vi "Drive Set Feet.vi"(1 "Feet":dbl=10.0 format="%#_13g", 2 "Direction":T1(ring)) -> (0 "Distance (ft)":dbl(knob) scale=0.0..10.0)   [LabVIEW 2014]
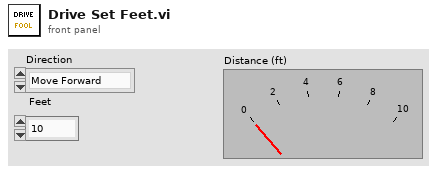
[diagram p1: front panel]
types:
  T1 = enum16{"Move Forward", "Move Backward", "Strafe Right", "Strafe Left"}
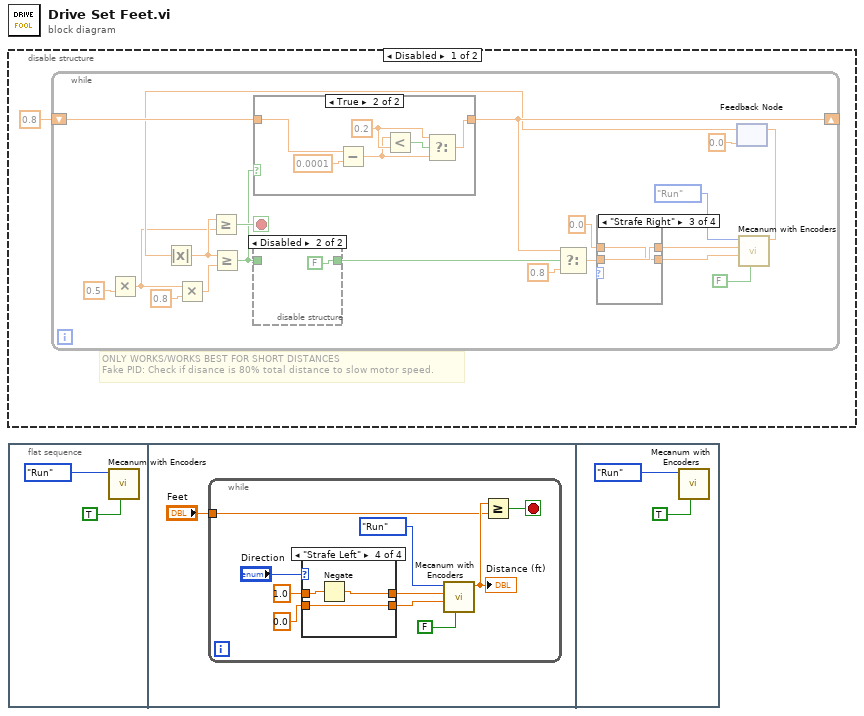
[diagram p0: block diagram]
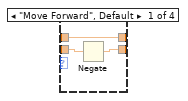
[diagram p4: hidden frame]
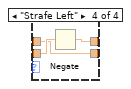
[diagram p6: hidden frame]
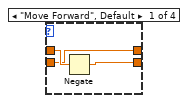
[diagram p8: hidden frame]
diagram:
  n1 = disable-structure shown="Disabled" {
    frame Disabled {
      # "ONLY WORKS/WORKS BEST FOR SHORT DISTANCES\nFake PID: Check if disance is 80% total distance to slow motor speed."
      n2 = while {
        shift-right: [w13] -> _
        shift-left: 0.8 -> [w14]
        stop <- w21 stop-if-true
        n3 = Multiply(y=0.5) -> (x*y=w3:dbl)  [unwired: 1 in]
        n4 = Multiply(x=w3, y=0.8) -> (x*y=w16:dbl)
        n5 = feedback #1(0.0 ("Distance (ft)")) -> (w7:dbl)
        n6 = Absolute Value(x=w7) -> (abs(x)=w6:dbl)
        n7 = Greater Or Equal?(x=w6, y=w3) -> (x >= y?=w21:bool)
        n8 = Greater Or Equal?(x=w6, y=w16) -> (x >= y?=w4:bool)
        n9 = case shown="True" w4 {
          tunnel: w14 -> [w24 w29]
          tunnel: [w24 w25] -> w13
          frame False {
          }
          frame True {
            w27 = 0.2 ("y")
            n10 = Subtract(x=w29, y=0.0001) -> (x-y=w26:dbl)
            n11 = Less?(x=w26, y=w27) -> (x < y?=w28:bool)
            n12 = Select(t=w27, s=w28, f=w26) -> (s? t:f=w25:dbl)
          }
        }
        n13 = disable-structure shown="Disabled" {
          disable-tunnel: [w22 FALSE] -> w5
          disable-tunnel: w4 -> [w22 _]
          frame Enabled {
          }
          frame Disabled {
          }
        }
        n14 = Select(t=w13, s=w5, f=0.8) -> (s? t:f=w12:dbl)
        n15 = case shown="\"Strafe Right\"" {
          selector: _ -> [_ _ _ _]
          tunnel: w12 -> [w32 w34 w37 w40]
          tunnel: [w31 w34 w36 w38] -> w20
          tunnel: [w33 w35 w37 w39] -> w19
          tunnel: 0.0 ("Turn") -> [w33 w35 w36 w38]
          frame "Move Forward", Default {
            n16 = Negate(x=w32) -> (-x=w31:dbl)
          }
          frame "Move Backward" {
          }
          frame "Strafe Right" {
          }
          frame "Strafe Left" {
            n17 = Negate(x=w40) -> (-x=w39:dbl)
          }
        }
        n18 = call "Mecanum with Encoders.vi"("Reset"=FALSE, "Forward/Backward"=w20, "Strafe"=w19, "Mode"=enum8{"Start", "Run", "Finish"}."Run") -> ("Distance (ft)"=w9:dbl)  [unwired: 6 in]
        n19 = feedback-in #1(w9) -> ()
      }
    }
    frame Enabled {
    }
  }
  n20 = flat-sequence {
    frame #0 {
      n21 = call "Mecanum with Encoders.vi"("Reset"=TRUE, "Mode"=enum8{"Start", "Run", "Finish"}."Run") -> ()  [unwired: 8 in, 1 out]
    }
    frame #1 {
      n22 = while {
        tunnel: "Feet" -> [w46]
        stop <- w45 stop-if-true
        n23 = case shown="\"Strafe Left\"" "Direction" {
          tunnel: [w54 w57 w59 w63] -> w51
          tunnel: 1.0 ("Strafe") -> [w56 w57 w60 w62]
          tunnel: [w55 w58 w60 w61] -> w49
          tunnel: 0.0 ("Strafe") -> [w55 w58 w59 w63]
          frame "Move Forward", Default {
            n24 = Negate(x=w56) -> (-x=w54:dbl)
          }
          frame "Move Backward" {
          }
          frame "Strafe Right" {
          }
          frame "Strafe Left" {
            n25 = Negate(x=w62) -> (-x=w61:dbl)
          }
        }
        n26 = call "Mecanum with Encoders.vi"("Reset"=FALSE, "Forward/Backward"=w51, "Strafe"=w49, "Mode"=enum8{"Start", "Run", "Finish"}."Run") -> ("Distance (ft)"=w47:dbl)  [unwired: 6 in]
        "Distance (ft)" <- w47
        n27 = Greater Or Equal?(x=w47, y=w46) -> (x >= y?=w45:bool)
      }
    }
    frame #2 {
      n28 = call "Mecanum with Encoders.vi"("Reset"=TRUE, "Mode"=enum8{"Start", "Run", "Finish"}."Run") -> ()  [unwired: 8 in, 1 out]
    }
  }
